vi "Actor Core.vi"(8 "error in":errorcluster, 11 "User Manager View In":refnum<class "User Manager View.lvclass">) -> (0 "error out":errorcluster, 3 "Actor out":refnum<class "Actor.lvclass">)   [LabVIEW 2017, in "User Manager View.lvlib" / "User Manager View.lvclass"]
doc: "(<B>Filename</B>: Actor Framework.lvlib:Actor.lvclass:Actor Core.vi)\n\nReceives messages to the actor, reacts to them, and initiates any error handling that may shut the actor down.\n\nDescendant classes may override this VI to append parallel tasks for the actor to complete while it handles messages. Overrides use the Call Parent Method node.\n\n<License>\nCopyright © 2017 Composed Systems, LLC | All rights reserved\nwww.composed.io\n\nAuthor: Ethan Stern <ethan.stern@composed.io>\n\nThis software is provided \"AS IS\" WITHOUT WARRANTIES, either express or implied, AND IS FOR EDUCATIONAL PURPOSES ONLY.\n</License>"
uses:
  <vilib>/gpm_packages/@cs/User Manager App/User Manager View/User Manager View/User Manager View.lvclass
  C:/Program Files/National Instruments/LabVIEW 2017/vi.lib/gpm_packages/@cs/mva-viewable/Source/ActorEvents/IEventAggregator/IEventAggregator.lvclass
  C:/Program Files/National Instruments/LabVIEW 2017/vi.lib/gpm_packages/@cs/mva-core/Source/IObserver/IObserver/IObserver.lvclass
  <vilib>/ActorFramework/Actor/Actor.lvclass
  <vilib>/gpm_packages/@cs/User Manager App/User Manager View/User Manager View Messages/Display All Users In Manager Msg/Display All Users In Manager Msg.lvclass
  C:/Program Files/National Instruments/LabVIEW 2017/vi.lib/gpm_packages/@cs/transport/Source/Concrete/ActorMessageTransport/Notification Msg/Notification Msg.lvclass
  <vilib>/event_ctls.llb/lveventtype.ctl
  <vilib>/gpm_packages/@cs/User Manager App/User Manager Model/Type Definitions/Credentials.ctl
  <vilib>/gpm_packages/@cs/User Manager App/User Manager Model/Type Definitions/User Levels.ctl
  <vilib>/gpm_packages/@cs/User Manager App/User Manager View/User Manager View Messages/Login Msg/Login Msg.lvclass
  <vilib>/gpm_packages/@cs/User Manager App/User Manager Model/Type Definitions/Successful Login Information.ctl
  <vilib>/gpm_packages/@cs/User Manager App/User Manager View/User Manager Type Defs/State.ctl
  <vilib>/gpm_packages/@cs/mva-core/Source/SubscriptionPolicy/BasicSubscription/BasicSubscription.lvclass/BasicSubscription.ctl
  <vilib>/gpm_packages/@cs/User Manager App/User Manager View/User Manager View/User Manager View.lvclass/User Manager View.ctl
  <vilib>/ActorFramework/Actor/Actor.lvclass/Actor.ctl
  <vilib>/ActorFramework/Message Enqueuer/Message Enqueuer.lvclass/Message Enqueuer.ctl
  <vilib>/gpm_packages/@cs/transport/Source/Concrete/ActorMessageTransport/ActorMessageTransport.lvclass/ActorMessageTransport.ctl
  <vilib>/gpm_packages/@cs/mva-core/Source/IMediator/SubscriptionRequest/SubscriptionRequest.lvclass/SubscriptionRequest.ctl
  <vilib>/gpm_packages/@cs/mva-core/Source/IObserver/IObserver Messages/Subscribe Msg/Subscribe Msg.lvclass/Subscribe Msg.ctl
  <vilib>/gpm_packages/@cs/mva-core/Source/IMediator/SubscriptionRequest/Pack Subscription Request.vi
  <vilib>/gpm_packages/@cs/mva-core/Source/IObserver/IObserver Messages/Subscribe Msg/Send Subscribe.vi
  <vilib>/ActorFramework/Actor/Read Self Enqueuer.vi
  <vilib>/gpm_packages/@cs/transport/Source/Concrete/ActorMessageTransport/Construct Actor Message Transport.vi
  <vilib>/ActorFramework/Message Enqueuer/Enqueue.vi
  <vilib>/ActorFramework/Message Enqueuer/Init from Existing Queue.vi
  <vilib>/ActorFramework/Message Enqueuer/Equals Not A Refnum.vi
  <vilib>/gpm_packages/@cs/mva-core/Source/SubscriptionPolicy/BasicSubscription/BasicSubscription.lvclass
  C:/Program Files/National Instruments/LabVIEW 2017/vi.lib/gpm_packages/@cs/mva-core/Source/IMediator/ISubscriptionPolicy/ISubscriptionPolicy.lvclass
  <vilib>/gpm_packages/@cs/mva-core/Source/IObserver/IObserver/IObserver.lvclass
  C:/Program Files/National Instruments/LabVIEW 2017/vi.lib/ActorFramework/Actor/Actor.lvclass
  <vilib>/gpm_packages/@cs/transport/Source/Concrete/ActorMessageTransport/ActorMessageTransport.lvclass
  C:/Program Files/National Instruments/LabVIEW 2017/vi.lib/gpm_packages/@cs/transport/Source/ITransport/ITransport.lvclass
  <vilib>/gpm_packages/@cs/mva-core/Source/IObserver/IObserver Messages/Subscribe Msg/Subscribe Msg.lvclass
  C:/Program Files/National Instruments/LabVIEW 2017/vi.lib/ActorFramework/Message/Message.lvclass
  <vilib>/Utility/error.llb/Error Cluster From Error Code.vi
  <vilib>/gpm_packages/@cs/mva-core/Source/IMediator/ISubscriptionPolicy/Open Subscription Policy.vi
  <vilib>/ActorFramework/Message Priority Queue/Priority Enqueue.vi
  <vilib>/ActorFramework/Message Enqueuer/Message Enqueuer.lvclass
  <vilib>/gpm_packages/@cs/mva-core/Source/IMediator/SubscriptionRequest/SubscriptionRequest.lvclass
  <vilib>/gpm_packages/@cs/transport/Source/Concrete/ActorMessageTransport/Notification Msg/Notification Msg.lvclass
  <vilib>/gpm_packages/@cs/mva-viewable/Source/IViewable/IViewable/IViewable.lvclass
  <vilib>/gpm_packages/@cs/mva-viewable/Source/ActorEvents/IEventAggregator/IEventAggregator.lvclass
  <vilib>/gpm_packages/@cs/User Manager App/User Manager Model/Type Definitions/User Manager Application Types.lvlib
  <vilib>/gpm_packages/@cs/User Manager App/User Manager View/User Manager View.lvlib
panel:
  in  "Undo":bool
  in  "User Information":T1
  in  "Save":bool
  in  "All Users":i32(listbox)
  in  "Remove":bool
  in  "Add User":bool
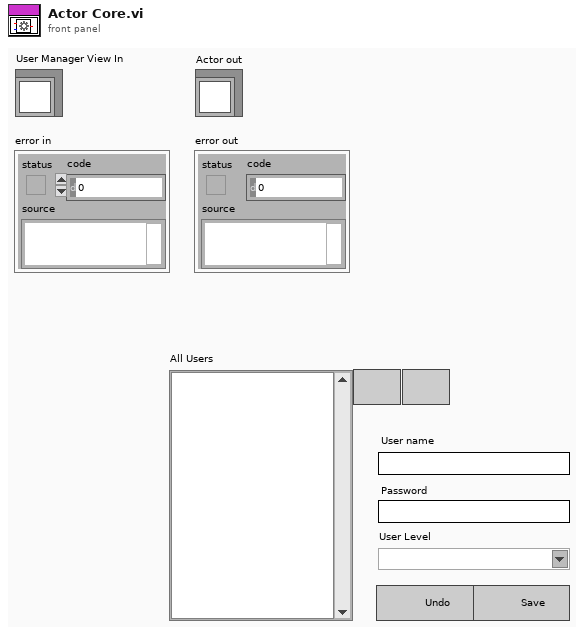
[diagram p1: front panel]
types:
  T1 = cluster{"User name":string, "Password":string, "User Level":string}
  T2 = typedef "User Manager View.lvlib/State.ctl" = enum16{"Normal", "Adding User", "Changing User Data"}
  T3 = typedef "User Manager Application Types.lvlib/Successful Login Information.ctl" = cluster{"Username":string, "User Level":T4, "User Levels In This Society":T4[]}
  T4 = typedef "User Manager Application Types.lvlib/User Levels.ctl" = cluster{"Rank":i32, "Title":string}
  T5 = typedef "User Manager Application Types.lvlib/Credentials.ctl" = cluster{"Username":string, "Password":string}
  T6 = typedef "lveventtype.ctl" = enum32{"Null", "Timeout", "Annotation Menu Selection", "Annotation Menu Selection?", "App Instance Close", "App Instance Close?", "Autoscale Range Change", "Bookmark Info Change", "Cell Edit", "Cell Edit?", "Cursor Grab", "Cursor Grab?", "Cursor Menu Selection", "Cursor Menu Selection?", "Cursor Move", "Cursor Release", "Data Change", "Direction Change", "Display State Change", "Drag Ended", "Drag Enter", "Drag Leave", "Drag Over", "Drag Source Update", "Drag Starting", "Drag Starting?", "Drop", "Exec State Change", "Key Down", "Key Down?", "Key Repeat", "Key Repeat?", "Key Up", "Listbox Double Click", "Menu Activation?", "Menu Selection (App)", "Menu Selection? (App)", "Menu Selection (User)", "Mouse Down", "Mouse Down?", "Mouse Enter", "Mouse Leave", "Mouse Move", "Mouse Up", "Mouse Wheel", "NI Security User Change (App)", "Pane Size", "Panel Close", "Panel Close?", "Panel Resize", "Plot Attribute Change", "Scale Range Change", "Shortcut Menu Activation?", "Shortcut Menu Selection (App)", "Shortcut Menu Selection? (App)", "Shortcut Menu Selection (User)", "Tree Double Click", "Tree Drag", "Tree Drag?", "Tree Drop", "Tree Drop?", "Tree Item Close", "Tree Item Close?", "Tree Item Open", "Tree Item Open?", "User Event", "Value Change"}
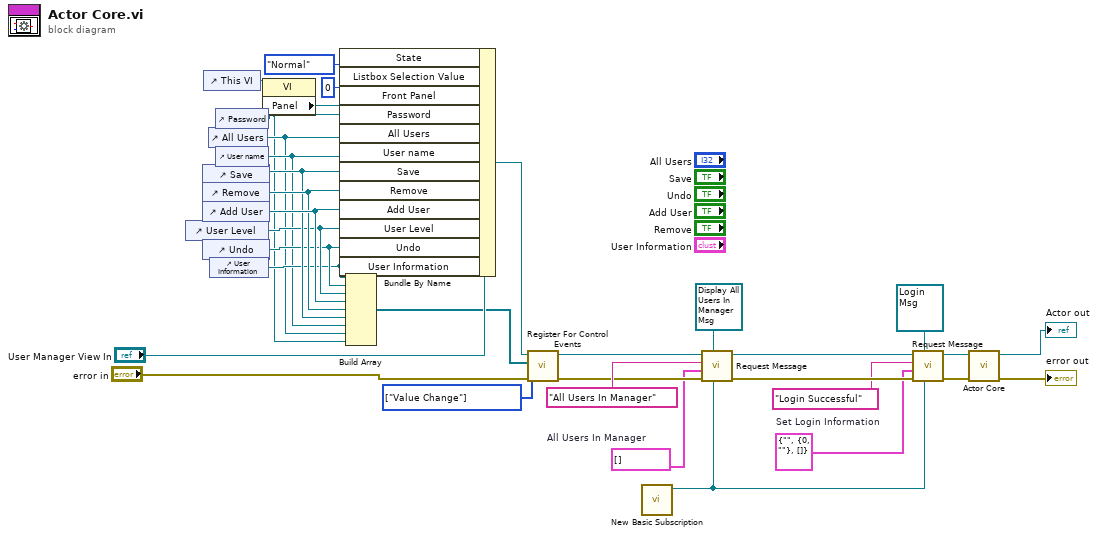
[diagram p0: block diagram]
diagram:
  w14 = T3 {"Username"="", "User Level"={"Rank"=0, "Title"=""}, "User Levels In This Society"=[]}  # Set Login Information
  w22 = cluster{"User Info":T5, "User Level":T4}[] []  # All Users In Manager
  w26 = T6[] [enum."Value Change"] items=["Null", "Timeout", "Annotation Menu Selection", "Annotation Menu Selection?", "App Instance Close", "App Instance Close?", "Autoscale Range Change", "Bookmark Info Change", "Cell Edit", "Cell Edit?", "Cursor Grab", "Cursor Grab?", "Cursor Menu Selection", "Cursor Menu Selection?", "Cursor Move", "Cursor Release", "Data Change", "Direction Change", "Display State Change", "Drag Ended", "Drag Enter", "Drag Leave", "Drag Over", "Drag Source Update", "Drag Starting", "Drag Starting?", "Drop", "Exec State Change", "Key Down", "Key Down?", "Key Repeat", "Key Repeat?", "Key Up", "Listbox Double Click", "Menu Activation?", "Menu Selection (App)", "Menu Selection? (App)", "Menu Selection (User)", "Mouse Down", "Mouse Down?", "Mouse Enter", "Mouse Leave", "Mouse Move", "Mouse Up", "Mouse Wheel", "NI Security User Change (App)", "Pane Size", "Panel Close", "Panel Close?", "Panel Resize", "Plot Attribute Change", "Scale Range Change", "Shortcut Menu Activation?", "Shortcut Menu Selection (App)", "Shortcut Menu Selection? (App)", "Shortcut Menu Selection (User)", "Tree Double Click", "Tree Drag", "Tree Drag?", "Tree Drop", "Tree Drop?", "Tree Item Close", "Tree Item Close?", "Tree Item Open", "Tree Item Open?", "User Event", "Value Change"] ("Registration Types")
  n1 = control-ref of="User Level"() -> (w6:refnum<vi>)
  n2 = control-ref of="Save"() -> (w7:refnum<vi>)
  n3 = control-ref of="Remove"() -> (w8:refnum<vi>)
  n4 = control-ref of="Add User"() -> (w9:refnum<vi>)
  n5 = control-ref of="Undo"() -> (w5:refnum<vi>)
  n6 = control-ref of="This VI"() -> (w21:refnum<vi>)
  n7 = control-ref of="All Users"() -> (w2:refnum<vi>)
  n8 = control-ref of="User Information"() -> (w4:refnum<vi>)
  n9 = control-ref of="Password"() -> (w1:refnum<vi>)
  n10 = control-ref of="User name"() -> (w3:refnum<vi>)
  n11 = property class="VI"(reference=w21) -> ("Panel"=w13:refnum<vi>)  [unwired: 1 in, 2 out]
  n12 = Bundle By Name(cluster="User Manager View In", "State"=State."Normal", "Listbox Selection Value"=0, "Front Panel"=w13, "Password"=w1, "All Users"=w2, "User name"=w3, "Save"=w7, "Remove"=w8, "Add User"=w9, "User Level"=w6, "Undo"=w5, "User Information"=w4) -> (w27:refnum<class "User Manager View.lvclass">)
  n13 = Build Array(w4, w5, w6, w9, w8, w7, w3, w2, w1) -> (w25:refnum<vi>[])
  n14 = call <vilib>:"Register For Control Events.vi"("error in (no error)"="error in", "Registration Types"=w26, "Control Refnums"=w25, "IEventAggregator In"=w27) -> ("error out"=w23:errorcluster, "IEventAggregator Out"=w24:refnum<class "User Manager View.lvclass">)  [unwired: 6 in]
  n15 = call <vilib>:"New Basic Subscription.vi"() -> ("BasicSubscription Out"=w17:refnum<class "BasicSubscription.lvclass">)  [unwired: 11 in]
  n16 = call <vilib>:"Request Message.vi"("Configured SubscriptionPolicy"=w17, "Desired Notification Msg"=refnum<class "Display All Users In Manager Msg.lvclass"> refnum ("User Manager View.lvlib:Display All Users In Manager Msg.lvclass"), "error in (no error)"=w23, "Data Type"=w22, "Datum Name"="All Users In Manager", "IObserver in"=w24) -> ("error out"=w19:errorcluster, "IObserver out"=w20:refnum<class "User Manager View.lvclass">)  [unwired: 3 in, 1 out]
  n17 = call <vilib>:"Request Message.vi"("Configured SubscriptionPolicy"=w17, "Desired Notification Msg"=refnum<class "Login Msg.lvclass"> refnum ("User Manager View.lvlib:Login Msg.lvclass"), "error in (no error)"=w19, "Data Type"=w14, "Datum Name"="Login Successful", "IObserver in"=w20) -> ("error out"=w18:errorcluster, "IObserver out"=w12:refnum<class "User Manager View.lvclass">)  [unwired: 3 in, 1 out]
  n18 = call-parent "Actor Core.vi"("error in"=w18, "IViewable In"=w12) -> ("error out"=→"error out":errorcluster, "Actor out"=→"Actor out":refnum<class "Actor.lvclass">)  [unwired: 8 in]
